vi "Read CFG File.vi"(8 "error in (no error)":errorcluster, 10 "File path":path, 11 "Mag Lab Measure Controller in":refnum<class "Mag Lab Measure Controller.lvclass">) -> (0 "error out":errorcluster, 3 "Mag Lab Measure Controller out":refnum<class "Mag Lab Measure Controller.lvclass">)   [LabVIEW 2015, in "Mag Lab Measure Controller.lvclass"]
uses:
  Mag Lab Measure Controller.lvclass
  Mag Lab Root Messages/Read CFG File Msg/Read CFG File Msg.lvclass/Read CFG File Msg.ctl
  <vilib>/ActorFramework/Message Enqueuer/Message Enqueuer.lvclass/Message Enqueuer.ctl
  <vilib>/ActorFramework/Message Enqueuer/Enqueue.vi
  <vilib>/ActorFramework/Message Priority Queue/Priority Enqueue.vi
  Mag Lab Root Messages/Read CFG File Msg/Read CFG File Msg.lvclass
  Mag Lab Measure Base/Mag Lab Measure Base.lvclass
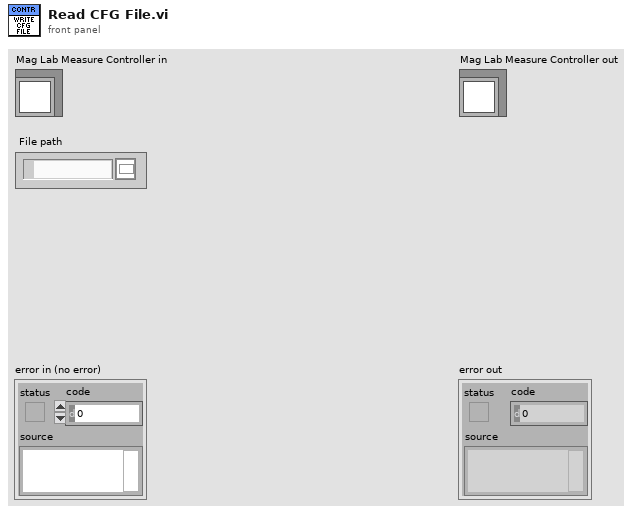
[diagram p1: front panel]
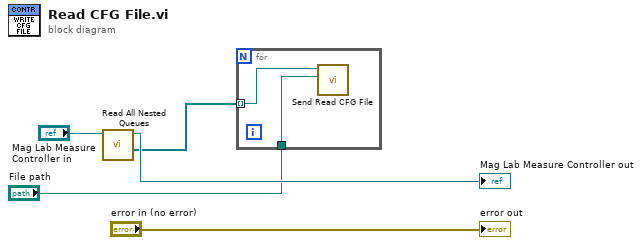
[diagram p0: block diagram]
diagram:
  n1 = call "Read All Nested Queues.vi"("Mag Lab Measure Base in"="Mag Lab Measure Controller in") -> ("Array of Queues"=w2:refnum<class "Message Enqueuer.lvclass">[], "Mag Lab Measure Base out"=→"Mag Lab Measure Controller out":refnum<class "Mag Lab Measure Controller.lvclass">)  [unwired: 7 in, 2 out]
  n2 = for {
    tunnel: w2 -> [w7] mode=indexing
    tunnel: "File path" -> [w6]
    n3 = call "Send Read CFG File.vi"("File path"=w6, "Message Enqueuer"=w7) -> ()  [unwired: 8 in, 2 out]
  }
  "error out" <- "error in (no error)"
